vi "Write Display Name.vi"(8 "error in (no error)":errorcluster, 10 "Display Name":string, 11 "Generic Node in":refnum<class "Generic Node.lvclass">) -> (0 "error out":errorcluster, 3 "Generic Node out":refnum<class "Generic Node.lvclass">)   [LabVIEW 2017, in "Browser Core.lvlib" / "Generic Node.lvclass"]
uses:
  Generic Node.lvclass
  Generic Node.lvclass/Generic Node.ctl
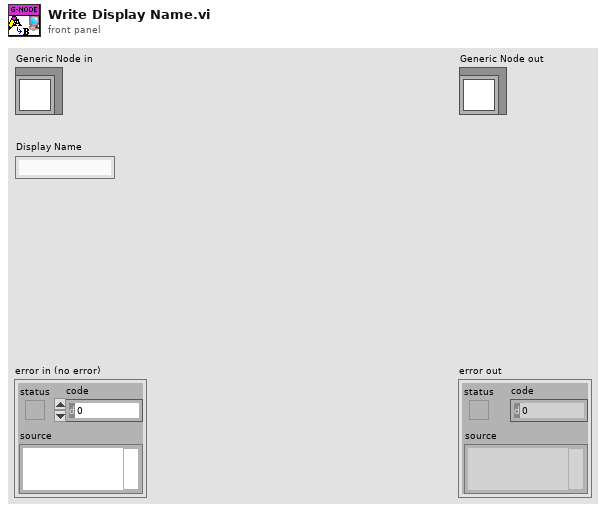
[diagram p1: front panel]
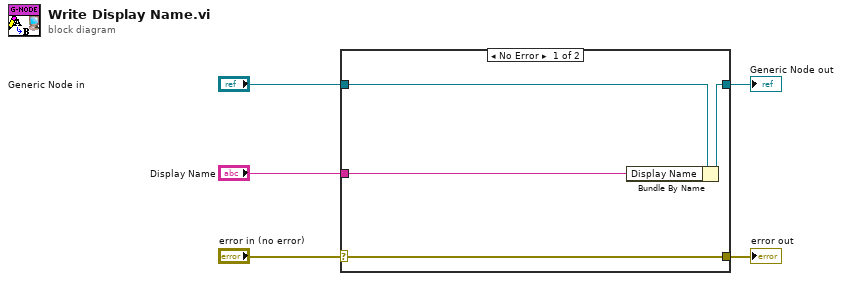
[diagram p0: block diagram]
diagram:
  n1 = case shown="No Error" "error in (no error)" {
    selector: "error in (no error)" -> [w9 w10]
    tunnel: [w9 w10] -> w4
    tunnel: [w7 w11] -> w2
    tunnel: "Generic Node in" -> [w8 w11]
    tunnel: "Display Name" -> [w6 _]
    frame No Error {
      n2 = Bundle By Name(cluster=w8, "Display Name"=w6) -> (w7:refnum<class "Generic Node.lvclass">)
    }
    frame Error {
    }
  }
  "error out" <- w4
  "Generic Node out" <- w2
